vi "proba.vi"() -> ()   [LabVIEW 2012]
uses:
  RosBridgeDotNet.dll
panel:
  in  "Ring":u16(ring)
  in  "Disconn":bool
  out "AktIP":string="10.2.5.194"
  in  "MelyIP":i32
  in  "Knob":dbl(knob)
  out "IPEredmeny":T1(array[cluster]) {"Status" items=["Success"=0, "DestinationNetworkUnreachable"=11002, "DestinationHostUnreachable"=11003, "DestinationProhibited, DestinationProtocolUnreachable"=11004, "DestinationPortUnreachable"=11005, "NoResources"=11006, "BadOption"=11007, "HardwareError"=11008, "PacketTooBig"=11009, "TimedOut"=11010, "BadRoute"=11012, "TtlExpired"=11013, "TtlReassemblyTimeExceeded"=11014, "ParameterProblem"=11015, "SourceQuench"=11016, "BadDestination"=11018, "DestinationUnreachable"=11040, "TimeExceeded"=11041, "BadHeader"=11042, "UnrecognizedNextHeader"=11043, "IcmpError"=11044, "DestinationScopeMismatch"=11045, "Unknown"=-1]}
  in  "Ping":bool
  in  "sebess":dbl[](array[numeric])
  in  "MessN":bool
  out "Error Out":errorcluster
  in  "MessT":bool
  in  "Connnect":bool
  in  "Array":T2(array[cluster])
  out "info":string
  out "XY Graph":cluster{dbl, dbl}[](graph)
  in  "_linear":dbl=1.0
  in  "_angular":dbl
  out "Connected":bool
  in  "Stop Button":bool
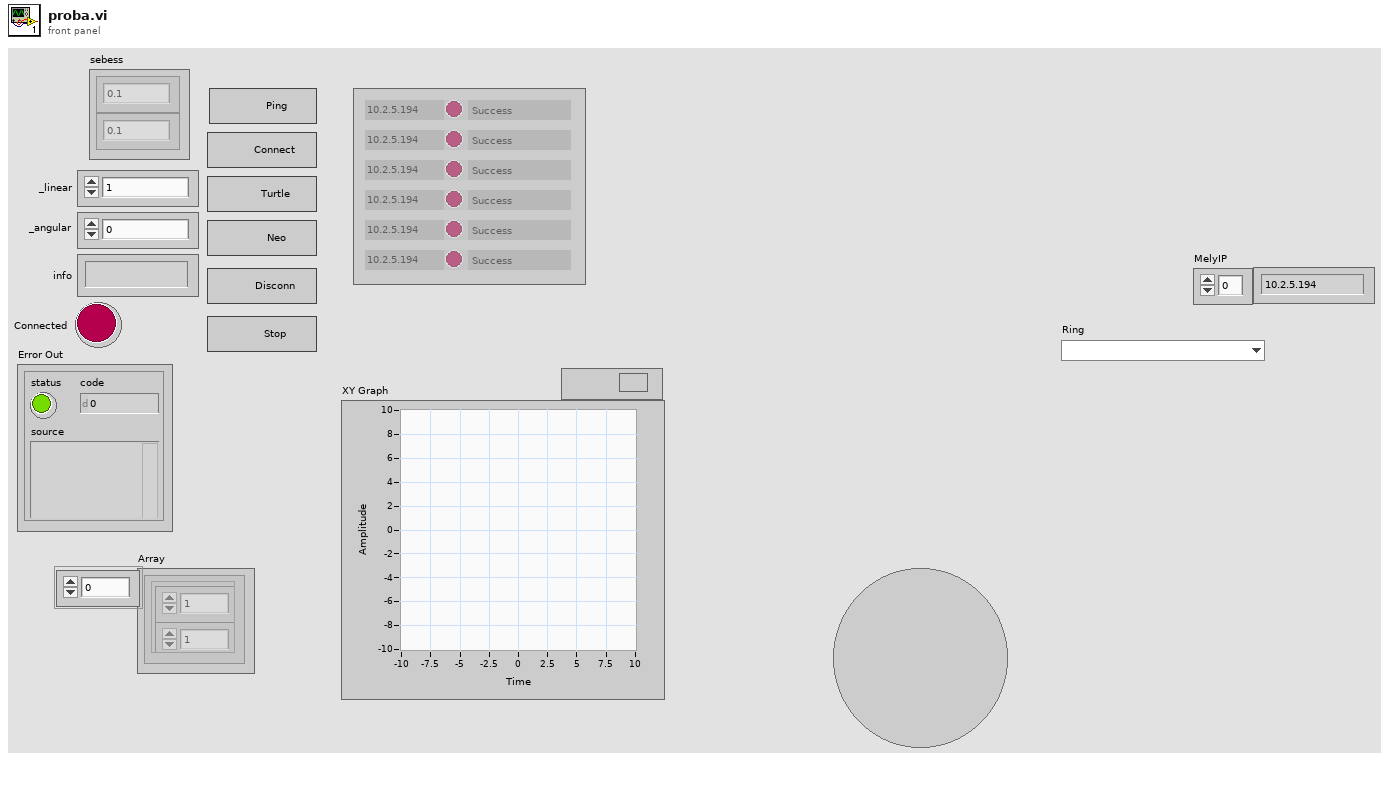
[diagram p1: front panel]
types:
  T1 = cluster{"pingelhet":bool, "IpAddress":string, "Status":i32}[]
  T2 = cluster{"Numeric Control":dbl, "Numeric Control 2":dbl}[]
  T3 = cluster{"pingelhet":bool, "IpAddress":string, "Status":i32}
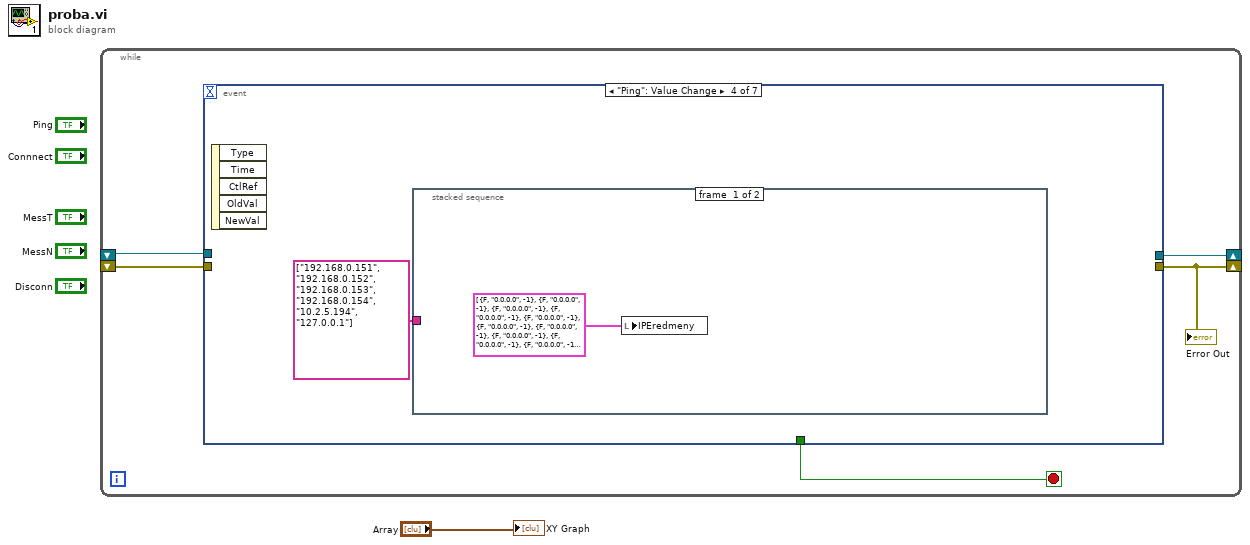
[diagram p0: block diagram]
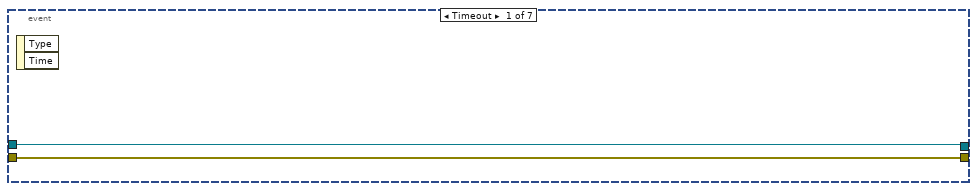
[diagram p2: hidden frame]
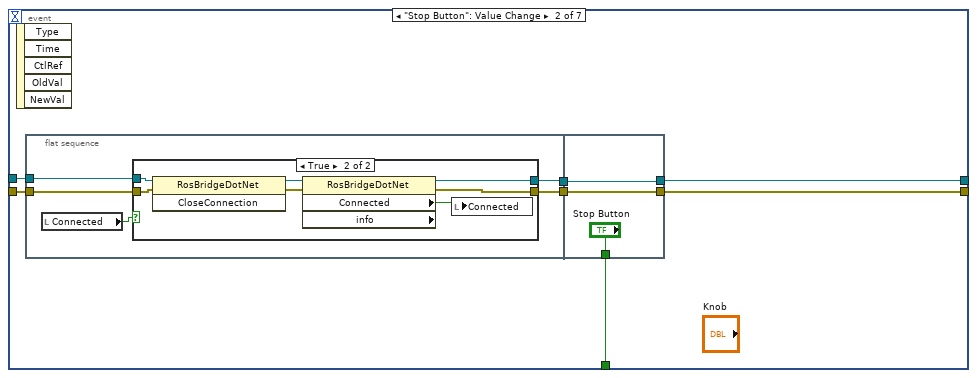
[diagram p3: hidden frame]
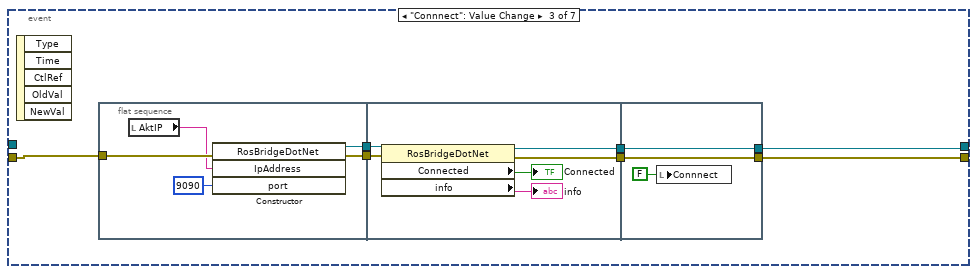
[diagram p5: hidden frame]
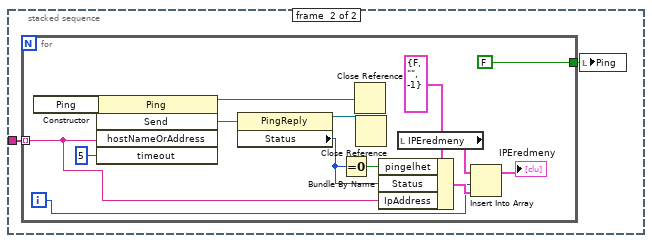
[diagram p6: hidden frame]
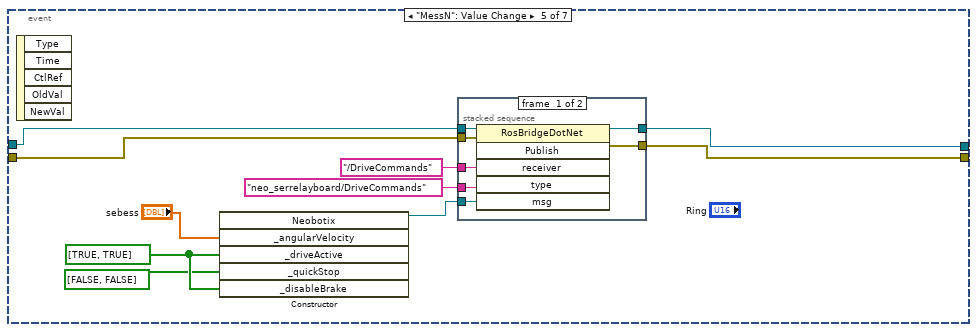
[diagram p7: hidden frame]
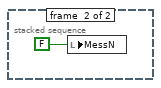
[diagram p8: hidden frame]
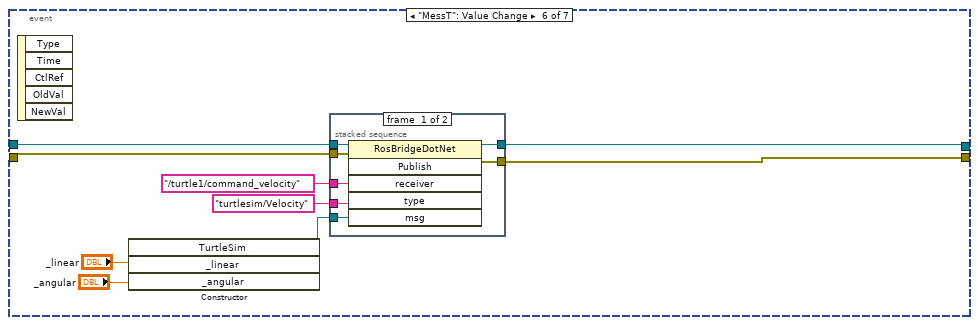
[diagram p9: hidden frame]
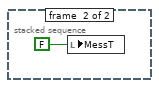
[diagram p10: hidden frame]
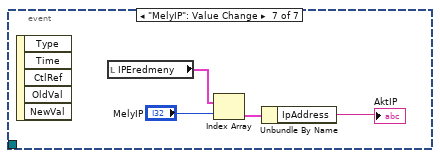
[diagram p11: hidden frame]
diagram:
  n1 = while {
    shift-right: [w5] -> _
    shift-left: _ -> [w3]
    shift-right: [w2] -> _
    shift-left: _ -> [w4]
    stop <- w6 stop-if-true
    n2 = event shown="[3] \"Ping\": Value Change" {
      selector: _ -> [_ _ _ _ _ _ _]
      dyn-events: _ -> [_ _ _ _ _ _ _]
      timeout: _ -> [_ _ _ _ _ _ _]
      tunnel: [_ w9 _ _ _ _ _] -> w6
      tunnel: [w8 w13 w33 _ w76 w91 _] -> w5
      tunnel: [w7 w12 w34 _ w75 w92 _] -> w2
      tunnel: w4 -> [w7 w14 w39 _ w77 w93 _]
      tunnel: w3 -> [w8 w15 _ _ w78 w90 _]
      event Timeout {
        n3 = event-data() -> ()  [unwired: 1 in, 2 out]
      }
      event "Stop Button": Value Change {
        n4 = event-data() -> ()  [unwired: 1 in, 5 out]
        n5 = flat-sequence {
          tunnel: w15 -> [w20]
          tunnel: w14 -> [w19]
          tunnel: [w18] -> w11
          tunnel: [w17] -> w10
          tunnel: [w31] -> w12
          tunnel: [w32] -> w13
          tunnel: w11 -> [w32]
          tunnel: w10 -> [w31]
          tunnel: ["Stop Button"] -> w9
          frame #0 {
            n6 = local read "Connected"() -> (w16:bool)
            n7 = case shown="True" w16 {
              tunnel: w20 -> [w22 w27]
              tunnel: w19 -> [w21 w26]
              tunnel: [w22 w25] -> w18
              tunnel: [w21 w24] -> w17
              frame False {
              }
              frame True {
                n8 = invoke class="RosBridgeDotNet" method="CloseConnection"(reference=w27, error in=w26) -> (reference out=w28:refnum<k24>, error out=w29:errorcluster)  [unwired: 1 in, 1 out]
                n9 = property class="RosBridgeDotNet" props=["Connected", "info"](reference=w28, error in=w29) -> (reference out=w25:refnum<k24>, error out=w24:errorcluster, "Connected"=w23:bool)  [unwired: 1 out]
                n10 = local write "Connected"(w23) -> ()
              }
            }
          }
          frame #1 {
          }
        }
      }
      event "Connnect": Value Change {
        n11 = event-data() -> ()  [unwired: 1 in, 5 out]
        n12 = flat-sequence {
          tunnel: [w43] -> w38
          tunnel: [w42] -> w37
          tunnel: w39 -> [w41]
          tunnel: w38 -> [w48]
          tunnel: w37 -> [w47]
          tunnel: [w46] -> w36
          tunnel: [w45] -> w35
          tunnel: w36 -> [w51]
          tunnel: w35 -> [w52]
          tunnel: [w52] -> w34
          tunnel: [w51] -> w33
          frame #0 {
            n13 = local read "AktIP"() -> (w40:string)
            n14 = constructor class="RosBridgeDotNet"(error in=w41, "IpAddress"=w40, "port"=9090) -> (reference out=w43:refnum<k24>, error out=w42:errorcluster)  [unwired: 2 in, 3 out]
          }
          frame #1 {
            n15 = property class="RosBridgeDotNet"(reference=w48, error in=w47) -> (reference out=w46:refnum<k24>, error out=w45:errorcluster, "Connected"=→"Connected":bool, "info"=→"info":string)
          }
          frame #2 {
            n16 = local write "Connnect"(FALSE ("Connnect")) -> ()
          }
        }
      }
      event "Ping": Value Change {
        n17 = event-data() -> ()  [unwired: 1 in, 5 out]
        n18 = stacked-sequence {
          tunnel: string[] ["192.168.0.151", "192.168.0.152", "192.168.0.153", "192.168.0.154", "10.2.5.194", "127.0.0.1"] ("IPCimek 3") -> [_ w56]
          frame #0 {
            n19 = local write "IPEredmeny"(T1 [{"pingelhet"=FALSE, "IpAddress"="0.0.0.0", "Status"=-1}, {"pingelhet"=FALSE, "IpAddress"="0.0.0.0", "Status"=-1}, {"pingelhet"=FALSE, "IpAddress"="0.0.0.0", "Status"=-1}, {"pingelhet"=FALSE, "IpAddress"="0.0.0.0", "Status"=-1}, {"pingelhet"=FALSE, "IpAddress"="0.0.0.0", "Status"=-1}, {"pingelhet"=FALSE, "IpAddress"="0.0.0.0", "Status"=-1}, {"pingelhet"=FALSE, "IpAddress"="0.0.0.0", "Status"=-1}, {"pingelhet"=FALSE, "IpAddress"="0.0.0.0", "Status"=-1}, {"pingelhet"=FALSE, "IpAddress"="0.0.0.0", "Status"=-1}, {"pingelhet"=FALSE, "IpAddress"="0.0.0.0", "Status"=-1}, {"pingelhet"=FALSE, "IpAddress"="0.0.0.0", "Status"=-1}] ("IPEredmeny 2")) -> ()
          }
          frame #1 {
            n20 = for {
              tunnel: [FALSE ("Ping")] -> w57
              tunnel: w56 -> [w61] mode=indexing
              i -> [w62]
              n21 = constructor class="Ping"() -> (reference out=w70:refnum<k24>)  [unwired: 3 in, 2 out]
              n22 = invoke class="Ping" method="Send"(reference=w70, "hostNameOrAddress"=w61, "timeout"=5) -> (reference out=w68:refnum<k24>, "Send"=w71:refnum<k24>)  [unwired: 2 in, 3 out]
              n23 = property class="PingReply"(reference=w71) -> (reference out=w69:refnum<k24>, "Status"=w66:i32)  [unwired: 1 in, 1 out]
              n24 = Equal To 0?(x=w66) -> (x = 0?=w59:bool)
              n25 = Close Reference(reference=w68) -> ()  [unwired: 1 in, 1 out]
              n26 = Close Reference(reference=w69) -> ()  [unwired: 1 in, 1 out]
              n27 = Bundle By Name(cluster=T3 {"pingelhet"=FALSE, "IpAddress"="", "Status"=-1} ("element"), "pingelhet"=w59, "Status"=w66, "IpAddress"=w61) -> (w63:T3)
              n28 = local read "IPEredmeny"() -> (w60:T1)
              n29 = Insert Into Array(array=w60, index=w62, new element=w63) -> (→"IPEredmeny":T1)
            }
            n30 = local write "Ping"(w57) -> ()
          }
        }
      }
      event "MessN": Value Change {
        w73 = bool[] [TRUE, TRUE] ("_driveActive")
        n31 = event-data() -> ()  [unwired: 1 in, 5 out]
        n32 = constructor class="RosBridgeDotNet+Neobotix"("_angularVelocity"="sebess", "_driveActive"=w73, "_quickStop"=bool[] [FALSE, FALSE] ("_driveActive"), "_disableBrake"=w73) -> (reference out=w79:refnum<k24>)  [unwired: 3 in, 6 out]
        n33 = stacked-sequence {
          tunnel: "/DriveCommands" ("receiver") -> [w88 _]
          tunnel: "neo_serrelayboard/DriveCommands" ("type") -> [w87 _]
          tunnel: w79 -> [w86 _]
          tunnel: w77 -> [w85 _]
          tunnel: [w84 _] -> w75
          tunnel: [w83 _] -> w76
          tunnel: w78 -> [w82 _]
          frame #0 {
            n34 = invoke class="RosBridgeDotNet" method="Publish"(reference=w82, error in=w85, "receiver"=w88, "type"=w87, "msg"=w86) -> (reference out=w83:refnum<k24>, error out=w84:errorcluster)  [unwired: 1 in, 4 out]
          }
          frame #1 {
            n35 = local write "MessN"(FALSE ("Message 2")) -> ()
          }
        }
      }
      event "MessT": Value Change {
        n36 = event-data() -> ()  [unwired: 1 in, 5 out]
        n37 = constructor class="RosBridgeDotNet+TurtleSim"("_linear"="_linear", "_angular"="_angular") -> (reference out=w94:refnum<k24>)  [unwired: 3 in, 4 out]
        n38 = stacked-sequence {
          tunnel: "/turtle1/command_velocity" ("receiver") -> [w105 _]
          tunnel: "turtlesim/Velocity" ("type") -> [w104 _]
          tunnel: w94 -> [w103 _]
          tunnel: w93 -> [w102 _]
          tunnel: [w101 _] -> w92
          tunnel: [w100 _] -> w91
          tunnel: w90 -> [w99 _]
          frame #0 {
            n39 = invoke class="RosBridgeDotNet" method="Publish"(reference=w99, error in=w102, "receiver"=w105, "type"=w104, "msg"=w103) -> (reference out=w100:refnum<k24>, error out=w101:errorcluster)  [unwired: 1 in, 4 out]
          }
          frame #1 {
            n40 = local write "MessT"(FALSE ("Message")) -> ()
          }
        }
      }
      event "MelyIP": Value Change {
        n41 = event-data() -> ()  [unwired: 1 in, 5 out]
        n42 = local read "IPEredmeny"() -> (w109:T1)
        n43 = Index Array(array=w109, index="MelyIP") -> (element=w108:T3)
        n44 = Unbundle By Name(w108) -> ("IpAddress"=→"AktIP":string)
      }
    }
    "Error Out" <- w2
  }
  "XY Graph" <- "Array"
